vi "Flush Shared Variable Data.vi"(8 "error in (no error)":errorcluster) -> (0 "error out":errorcluster)   [LabVIEW 2020, in "NI_VariableUtilities.lvlib"]
doc: "Flushes the buffer of all network-published shared variables immediately. LabVIEW uses an 8 kilobyte buffer for all shared variable values, and LabVIEW automatically flushes the 8 kilobyte buffer either when the buffer fills up or after 10 ms have passed."
uses:
  <vilib>/Utility/Variable/NI_VariableUtilities.lvlib
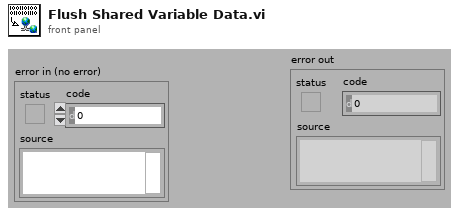
[diagram p1: front panel]
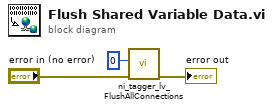
[diagram p0: block diagram]
diagram:
  n1 = call <vilib>:"ni_tagger_lv_FlushAllConnections.vi"("error in (no error)"="error in (no error)", "timeout ms (1000)"=0) -> ("error out"=→"error out":errorcluster)  [unwired: 8 in, 1 out]
